vi "alg_eigenValues (SubVI).vi"(8 "에러 입력(에러 없음)":errorcluster, 11 "matrix":dbl[][](array[numeric])=[[1.0, 2.0], [3.0, 4.0]]) -> (0 "에러 출력":errorcluster, 1 "Eigen values":cdb[](array[numeric]) caption="고유값", 2 "Eigen vectors":cdb[][](array[numeric]), 3 "참조 번호 출력":refnum<k35>)   [LabVIEW 2018]
uses:
  PythonConfigGlobal.vi
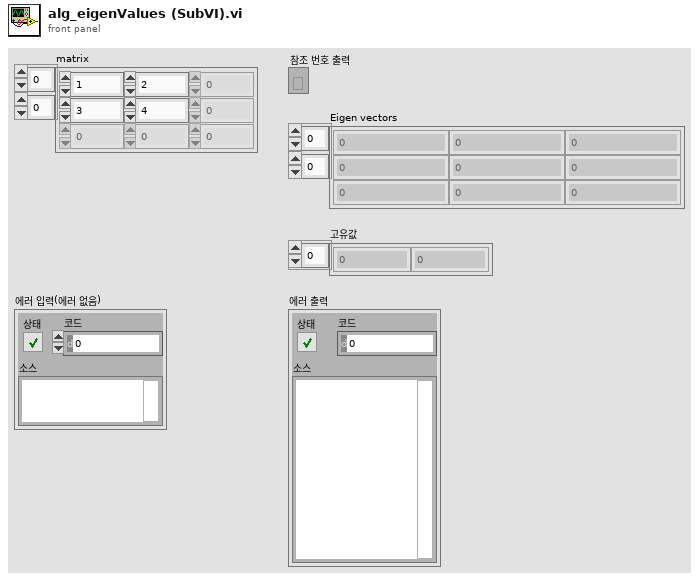
[diagram p1: front panel]
types:
  T1 = cluster{"session out":refnum<k35>, "appended path":path}
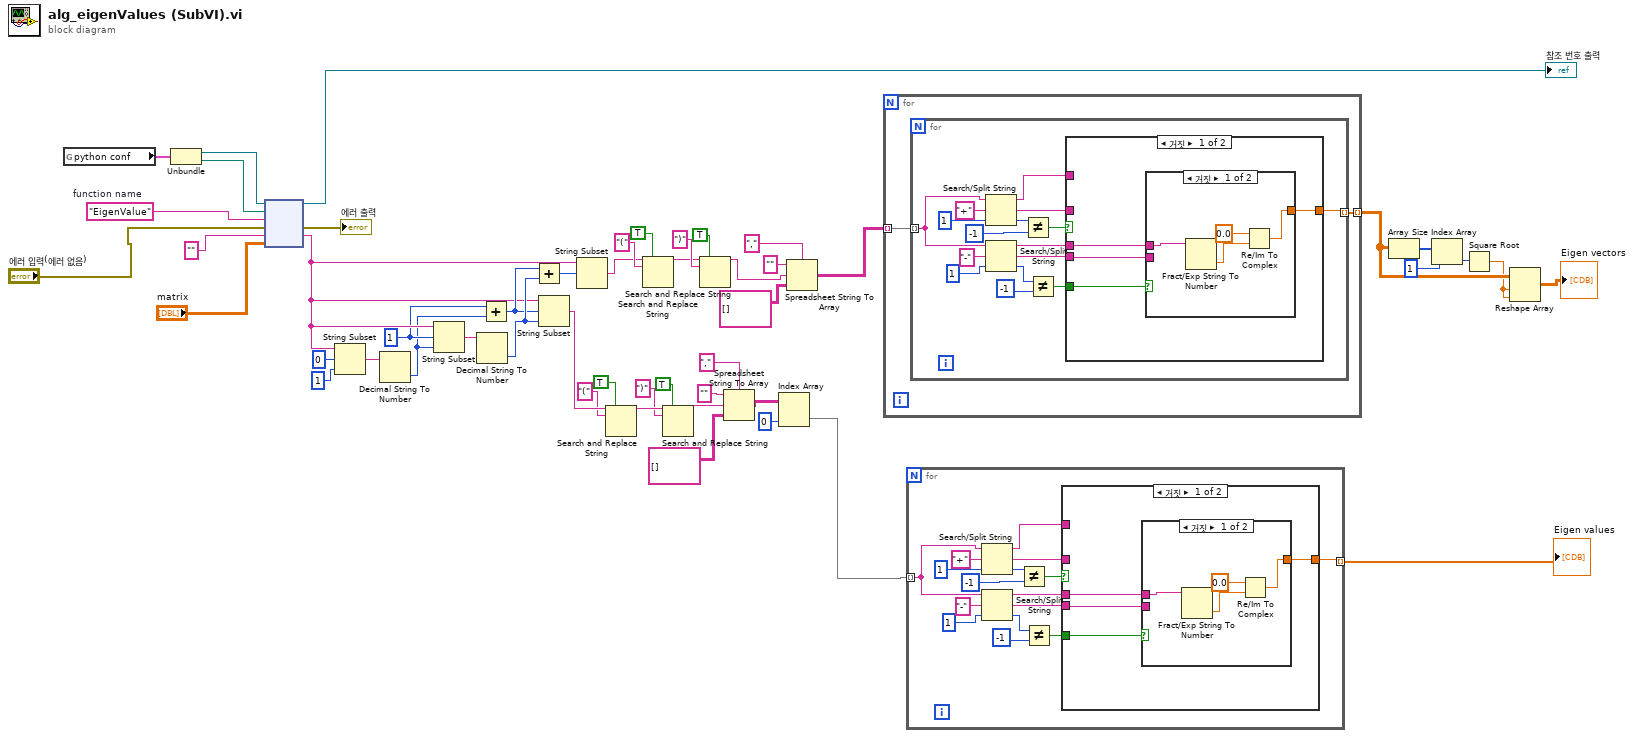
[diagram p0: block diagram]
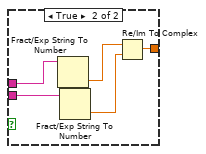
[diagram p2: hidden frame]
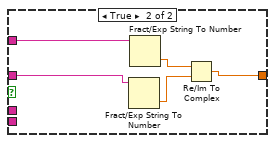
[diagram p3: hidden frame]
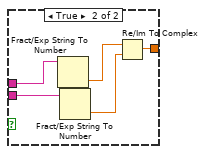
[diagram p4: hidden frame]
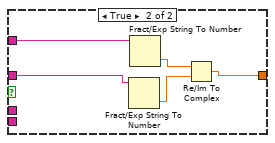
[diagram p5: hidden frame]
diagram:
  w14 = 1 ("오프셋(0)")
  w2 = "EigenValue"  # function name
  n1 = global read "PythonConfigGlobal.vi" "python conf"() -> (w5:T1)
  n2 = Unbundle(w5) -> ("session out"=w3:refnum<k35>, "appended path"=w4:path)
  n3 = node(w3, w4, w2, "에러 입력(에러 없음)", "", "matrix") -> (→"참조 번호 출력":refnum<k35>, →"에러 출력":errorcluster, w15:string)  [unwired: 1 in, 2 out]
  n4 = String Subset(string=w15, offset (0)=0 ("오프셋(0)"), length (rest)=1 ("길이(나머지)")) -> (substring=w11:string)
  n5 = Decimal String To Number(string=w11) -> (number=w13:i32)  [unwired: 2 in, 1 out]
  n6 = String Subset(string=w15, offset (0)=w14, length (rest)=w13) -> (substring=w12:string)
  n7 = Decimal String To Number(string=w12) -> (number=w17:i32)  [unwired: 2 in, 1 out]
  n8 = Add(x=w14, y=w13) -> (x+y=w16:i32)
  n9 = Add(x=w16, y=w17) -> (x+y=w18:i32)
  n10 = String Subset(string=w15, offset (0)=w16, length (rest)=w17) -> (substring=w50:string)
  n11 = String Subset(string=w15, offset (0)=w18) -> (substring=w35:string)  [unwired: 1 in]
  n12 = Search and Replace String(replace all?=TRUE ("모두 대체? (거짓)"), input string=w50, search string="(" ("검색 문자열")) -> (result string=w47:string)  [unwired: 5 in, 3 out]
  n13 = Search and Replace String(replace all?=TRUE ("모두 대체? (거짓)"), input string=w35, search string="(" ("검색 문자열")) -> (result string=w37:string)  [unwired: 5 in, 3 out]
  n14 = Search and Replace String(replace all?=TRUE ("모두 대체? (거짓)"), input string=w47, search string=")" ("검색 문자열")) -> (result string=w49:string)  [unwired: 5 in, 3 out]
  n15 = Search and Replace String(replace all?=TRUE ("모두 대체? (거짓)"), input string=w37, search string=")" ("검색 문자열")) -> (result string=w39:string)  [unwired: 5 in, 3 out]
  n16 = Spreadsheet String To Array(delimiter (Tab)="," ("구분 문자 (탭)"), format string="" ("포맷 문자열"), spreadsheet string=w49, array type (2D Dbl)=string[][] [] ("배열 타입(2D Dbl)")) -> (array=w26:string[][])
  n17 = Index Array(array=w26, index (row)=0 ("인덱스 (행)")) -> (element=w42:string[])  [unwired: 1 in]
  n18 = Spreadsheet String To Array(delimiter (Tab)="," ("구분 문자 (탭)"), format string="" ("포맷 문자열"), spreadsheet string=w39, array type (2D Dbl)=string[][] [] ("배열 타입(2D Dbl)")) -> (array=w32:string[][])
  n19 = for {
    tunnel: w32 -> [w52] mode=indexing
    tunnel: [w51] -> w33 mode=indexing
    n20 = for {
      tunnel: w52 -> [w53] mode=indexing
      tunnel: [w54] -> w51 mode=indexing
      n21 = Search/Split String(string=w53, search string/char (-)="+" ("검색 문자열"), offset (0)=1 ("오프셋(0)")) -> (substring before match=w63:string, match + rest of string=w62:string, offset of match=w66:i32)
      n22 = Search/Split String(string=w53, search string/char (-)="-" ("검색 문자열"), offset (0)=1 ("오프셋(0)")) -> (substring before match=w60:string, match + rest of string=w61:string, offset of match=w57:i32)
      n23 = Not Equal?(x=w66, y=-1) -> (x != y?=w64:bool)
      n24 = Not Equal?(x=w57, y=-1) -> (x != y?=w55:bool)
      n25 = case shown="거짓" w64 {
        tunnel: w63 -> [_ w86]
        tunnel: w62 -> [_ w85]
        tunnel: [w70 w82] -> w54
        tunnel: w61 -> [w72 _]
        tunnel: w60 -> [w71 _]
        tunnel: w55 -> [w69 _]
        frame False {
          n26 = case shown="거짓" w69 {
            tunnel: w72 -> [_ w79]
            tunnel: w71 -> [w76 w78]
            tunnel: [w73 w77] -> w70
            frame False {
              n27 = Fract/Exp String To Number(string=w76) -> (number=w75:dbl)  [unwired: 3 in, 1 out]
              n28 = Re/Im To Complex(1:w75, 2:0.0 ("x")) -> (0:w73:cdb)
            }
            frame True {
              n29 = Fract/Exp String To Number(string=w78) -> (number=w81:dbl)  [unwired: 3 in, 1 out]
              n30 = Fract/Exp String To Number(string=w79) -> (number=w80:dbl)  [unwired: 3 in, 1 out]
              n31 = Re/Im To Complex(1:w80, 2:w81) -> (0:w77:cdb)
            }
          }
        }
        frame True {
          n32 = Fract/Exp String To Number(string=w85) -> (number=w83:dbl)  [unwired: 3 in, 1 out]
          n33 = Fract/Exp String To Number(string=w86) -> (number=w84:dbl)  [unwired: 3 in, 1 out]
          n34 = Re/Im To Complex(1:w83, 2:w84) -> (0:w82:cdb)
        }
      }
    }
  }
  n35 = for {
    tunnel: w42 -> [w87] mode=indexing
    tunnel: [w88] -> w43 mode=indexing
    n36 = Search/Split String(string=w87, search string/char (-)="+" ("검색 문자열"), offset (0)=1 ("오프셋(0)")) -> (substring before match=w97:string, match + rest of string=w96:string, offset of match=w100:i32)
    n37 = Search/Split String(string=w87, search string/char (-)="-" ("검색 문자열"), offset (0)=1 ("오프셋(0)")) -> (substring before match=w94:string, match + rest of string=w95:string, offset of match=w91:i32)
    n38 = Not Equal?(x=w100, y=-1) -> (x != y?=w98:bool)
    n39 = Not Equal?(x=w91, y=-1) -> (x != y?=w89:bool)
    n40 = case shown="거짓" w98 {
      tunnel: w97 -> [_ w120]
      tunnel: w96 -> [_ w119]
      tunnel: [w104 w116] -> w88
      tunnel: w95 -> [w106 _]
      tunnel: w94 -> [w105 _]
      tunnel: w89 -> [w103 _]
      frame False {
        n41 = case shown="거짓" w103 {
          tunnel: w106 -> [_ w113]
          tunnel: w105 -> [w110 w112]
          tunnel: [w107 w111] -> w104
          frame False {
            n42 = Fract/Exp String To Number(string=w110) -> (number=w109:dbl)  [unwired: 3 in, 1 out]
            n43 = Re/Im To Complex(1:w109, 2:0.0 ("x")) -> (0:w107:cdb)
          }
          frame True {
            n44 = Fract/Exp String To Number(string=w112) -> (number=w115:dbl)  [unwired: 3 in, 1 out]
            n45 = Fract/Exp String To Number(string=w113) -> (number=w114:dbl)  [unwired: 3 in, 1 out]
            n46 = Re/Im To Complex(1:w114, 2:w115) -> (0:w111:cdb)
          }
        }
      }
      frame True {
        n47 = Fract/Exp String To Number(string=w119) -> (number=w117:dbl)  [unwired: 3 in, 1 out]
        n48 = Fract/Exp String To Number(string=w120) -> (number=w118:dbl)  [unwired: 3 in, 1 out]
        n49 = Re/Im To Complex(1:w117, 2:w118) -> (0:w116:cdb)
      }
    }
  }
  "Eigen values" <- w43
  n50 = Array Size(array=w33) -> (size(s)=w21:i32[])
  n51 = Index Array(array=w21, index=1 ("인덱스")) -> (element=w22:i32)
  n52 = Square Root(x=w22) -> (sqrt(x)=w24:dbl)
  n53 = Reshape Array(w33, w24, w24) -> (→"Eigen vectors":cdb[][])
